vi "Intake Ramp.vi"(10 "Intake":bool, 11 "Outtake":bool) -> ()   [LabVIEW 2016]
uses:
  <vilib>/Rock Robotics/WPI/ThirdParty/CanMotor/TalonSRX/WPI_CANTalonSRX_BrakeOverride.ctl
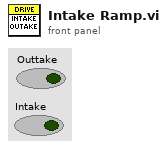
[diagram p1: front panel]
types:
  T1 = typedef "WPI_CANTalonSRX_BrakeOverride.ctl" = enum8{"No Override", "Override to Coast", "Override to Brake"}
  T2 = typedef "WPI_MotorControlDeviceRef.ctl" = cluster{"DeviceStatus":errorcluster, "Type":T3, "PWM":cluster{"PWM Channel":T4, "DeadBand":T5}, "CAN":cluster{"Device Number":u8, "SetOutput VI Ref":variant, "GetOutput VI Ref":variant, "Enable VI Ref":variant, "Disable VI Ref":variant, "Data":variant}, "Invert":bool}
  T3 = typedef "WPI_MotorControlType.ctl" = enum16{"PWM", "CAN"}
  T4 = typedef "FPGA_DIOPWMChannel.ctl" = enum8{"PWM 0", "PWM 1", "PWM 2", "PWM 3", "PWM 4", "PWM 5", "PWM 6", "PWM 7", "PWM 8", "PWM 9", "PWM MXP 0", "PWM MXP 1", "PWM MXP 2", "PWM MXP 3", "PWM MXP 4", "PWM MXP 5", "PWM MXP 6", "PWM MXP 7", "PWM MXP 8", "PWM MXP 9", "Invalid"}
  T5 = typedef "WPI_PWMDeadband.ctl" = cluster{"Name":string, "maxPositivePwm":i32, "minPositivePwm":i32, "centerPwm":i32, "maxNegativePwm":i32, "minNegativePwm":i32, "angularRange":u16}
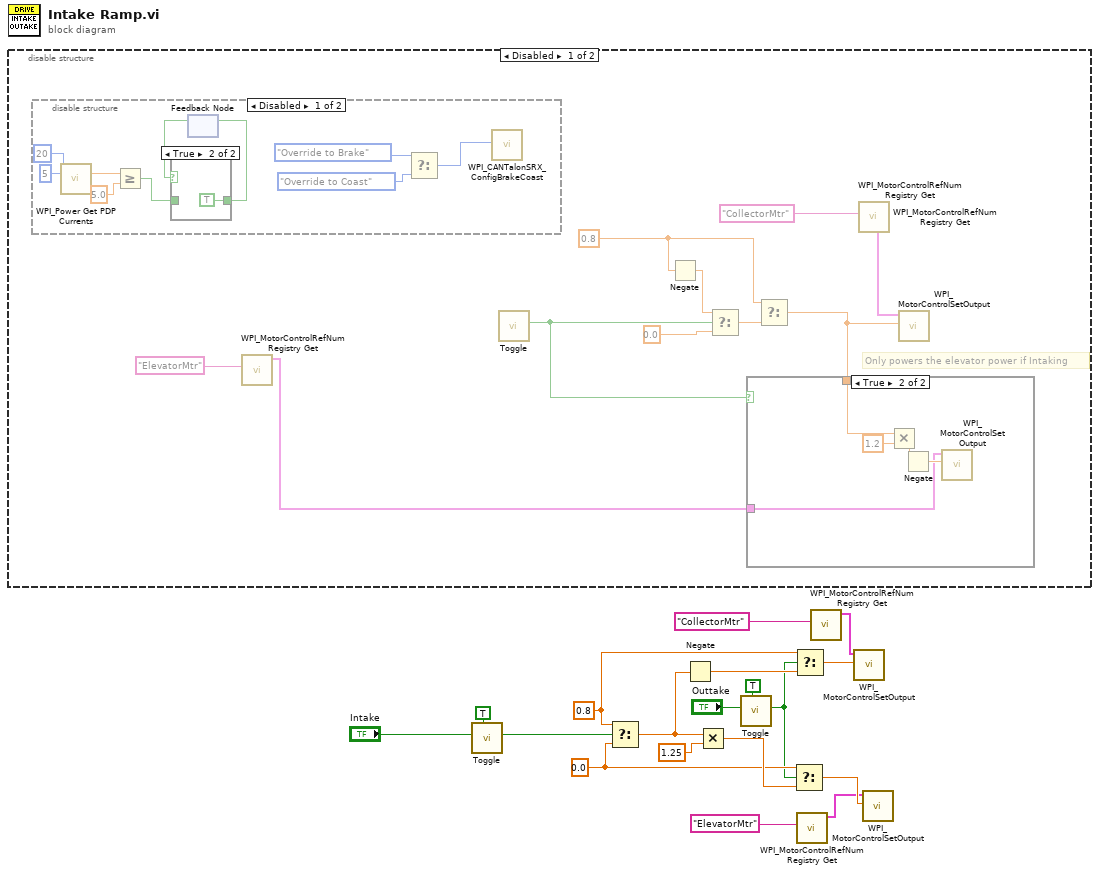
[diagram p0: block diagram]
diagram:
  w11 = 0.8 ("t")
  w10 = 0.0 ("f")
  n1 = disable-structure shown="Disabled" {
    frame Disabled {
      w20 = 0.8 ("x")
      # "Only powers the elevator power if Intaking"
      n2 = disable-structure shown="Disabled" {
        frame Disabled {
          n3 = call <vilib>:"WPI_Power Get PDP Currents.vi"("Power Distribution Panel (0)"=u8 20, "PDP Channel"=5) -> ("current (A)"=w38:dbl)  [unwired: 11 in, 2 out]
          n4 = Greater Or Equal?(x=w38, y=5.0) -> (x >= y?=w36:bool)
          n5 = feedback #1() -> (w34:bool)  [unwired: 1 in]
          n6 = case shown="True" w34 {
            tunnel: w36 -> [w41 _]
            tunnel: [w41 TRUE] -> w35
            frame False {
            }
            frame True {
            }
          }
          n7 = feedback-in #1(w35) -> ()
          n8 = Select(t=WPI_CANTalonSRX_BrakeOverride."Override to Brake" ("Brake / Coast Mode"), f=WPI_CANTalonSRX_BrakeOverride."Override to Coast" ("Brake / Coast Mode")) -> (s? t:f=w33:T1)  [unwired: 1 in]
          n9 = call <vilib>:"WPI_CANTalonSRX_ConfigBrakeCoast.vi"("Brake / Coast Mode"=w33) -> ()  [unwired: 9 in, 2 out]
        }
        frame Enabled {
        }
      }
      n10 = call <vilib>:"WPI_MotorControlRefNum Registry Get.vi"("refnum name"="ElevatorMtr") -> ("MotorControlDevRef"=w21:T2)  [unwired: 9 in, 1 out]
      n11 = call "Toggle.vi"() -> ("Output"=w23:bool)  [unwired: 11 in]
      n12 = Negate(x=w20) -> (-x=w30:dbl)
      n13 = Select(t=w30, s=w23, f=0.0) -> (s? t:f=w29:dbl)
      n14 = Select(t=w20, f=w29) -> (s=w25:bool, s? t:f=w24:dbl)
      n15 = case shown="True" w23 {
        tunnel: w24 -> [_ w43]
        tunnel: w21 -> [_ w44]
        frame False {
        }
        frame True {
          n16 = Multiply(x=w43, y=1.2) -> (x*y=w45:dbl)
          n17 = Negate(x=w45) -> (-x=w47:dbl)
          n18 = call <vilib>:"WPI_MotorControlSetOutput.vi"("Output"=w47, "MotorControlDevRef"=w44) -> ()  [unwired: 7 in, 3 out]
        }
      }
      n19 = call <vilib>:"WPI_MotorControlRefNum Registry Get.vi"("refnum name"="CollectorMtr") -> ()  [unwired: 9 in, 2 out]
      n20 = call <vilib>:"WPI_MotorControlRefNum Registry Get.vi"("refnum name"="CollectorMtr") -> ("MotorControlDevRef"=w27:T2)  [unwired: 9 in, 1 out]
      n21 = call <vilib>:"WPI_MotorControlSetOutput.vi"("Output"=w24, "MotorControlDevRef"=w27) -> ()  [unwired: 7 in, 3 out]
    }
    frame Enabled {
    }
  }
  n22 = call "Toggle.vi"("Control"=TRUE, "Input"="Intake") -> ("Output"=w18:bool)  [unwired: 9 in]
  n23 = Select(t=w11, s=w18, f=w10) -> (s? t:f=w16:dbl)
  n24 = Negate(x=w16) -> (-x=w15:dbl)
  n25 = Multiply(x=w16, y=1.25) -> (x*y=w14:dbl)
  n26 = call "Toggle.vi"("Control"=TRUE, "Input"="Outtake") -> ("Output"=w2:bool)  [unwired: 9 in]
  n27 = Select(t=w10, s=w2, f=w14) -> (s? t:f=w12:dbl)
  n28 = Select(t=w11, s=w2, f=w15) -> (s? t:f=w13:dbl)
  n29 = call <vilib>:"WPI_MotorControlRefNum Registry Get.vi"("refnum name"="ElevatorMtr") -> ("MotorControlDevRef"=w7:T2)  [unwired: 9 in, 1 out]
  n30 = call <vilib>:"WPI_MotorControlRefNum Registry Get.vi"("refnum name"="CollectorMtr") -> ("MotorControlDevRef"=w5:T2)  [unwired: 9 in, 1 out]
  n31 = call <vilib>:"WPI_MotorControlSetOutput.vi"("Output"=w13, "MotorControlDevRef"=w5) -> ()  [unwired: 7 in, 3 out]
  n32 = call <vilib>:"WPI_MotorControlSetOutput.vi"("Output"=w12, "MotorControlDevRef"=w7) -> ()  [unwired: 7 in, 3 out]
